vi "Time Trace.vi"() -> ()   [LabVIEW 2011]
uses:
  <vilib>/DAQmx/read.llb/DAQmx Read (Counter U32 1Chan 1Samp).vi
  <vilib>/DAQmx/create/channels.llb/DAQmx Create Channel (CI-Count Edges).vi
  <vilib>/DAQmx/configure/timing.llb/DAQmx Timing (Sample Clock).vi
  <vilib>/DAQmx/miscellaneous.llb/DAQmx Fill In Error Info.vi
  <vilib>/Utility/file.llb/Write To Spreadsheet File (DBL).vi
  Program Files/National Instruments/LabVIEW 2011/resource/objmgr/daqmx.rc
panel:
  in  "Save?":bool
  in  "file path (dialog if empty)":path
  out "XY Graph":cluster{"Y":dbl[], "Y":dbl[]}[](graph)
  in  "Time Target (s)":dbl=1.0
  in  "stop":bool
  in  "rate (Hz)":dbl=1000.0 format="%0.2f"
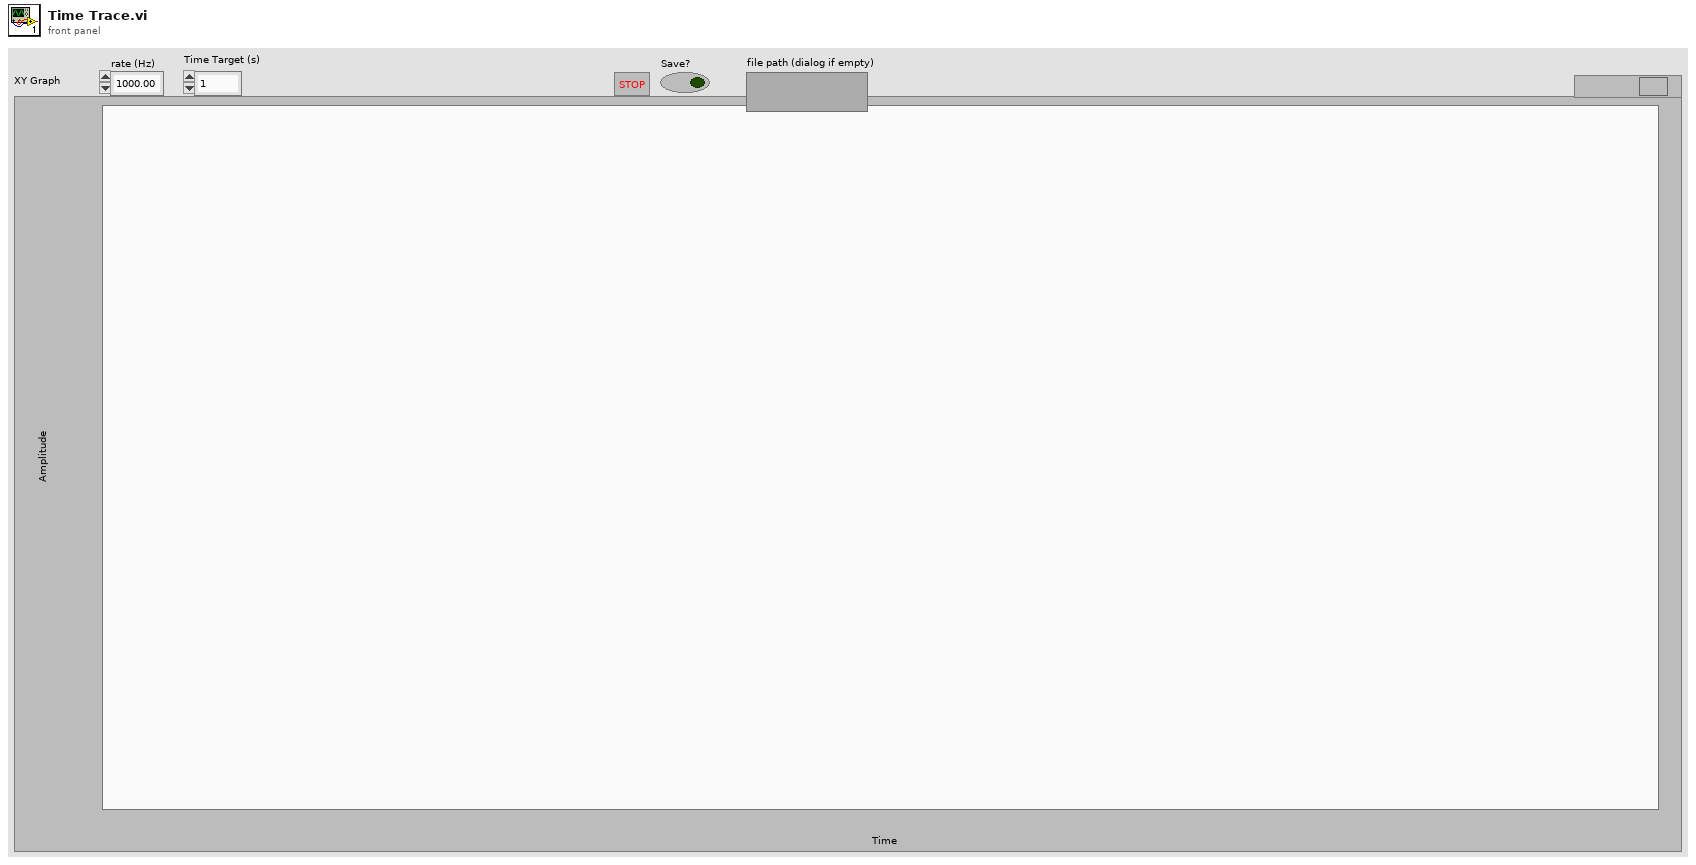
[diagram p1: front panel]
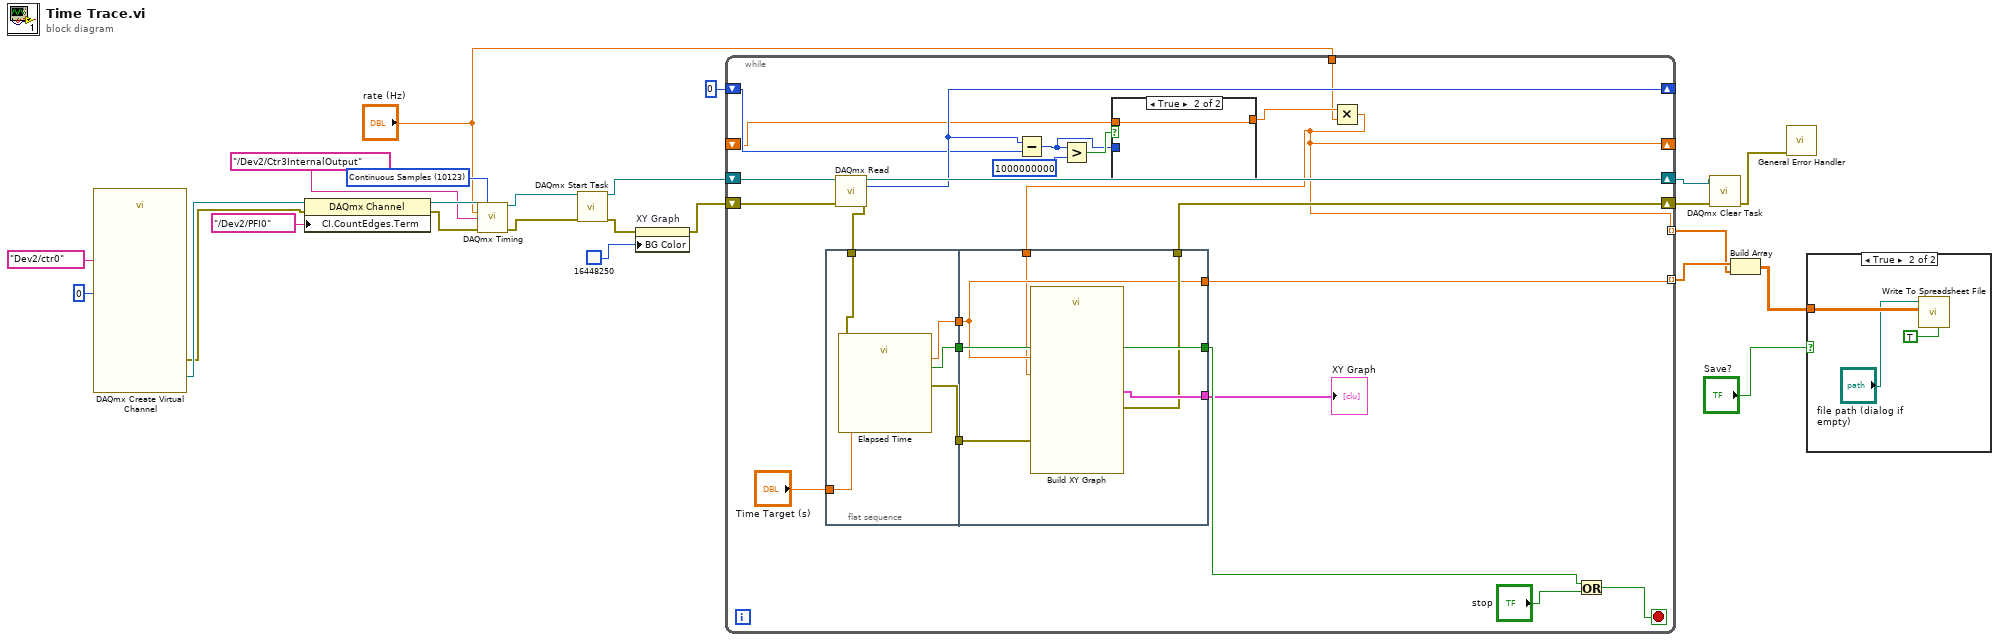
[diagram p0: block diagram]
diagram:
  w4 = 10123 items=["Finite Samples"=10178, "Continuous Samples"=10123, "Hardware Timed Single Point"=12522] ("sample mode")
  n1 = call-poly <vilib>:"DAQmx Create Virtual Channel.vi"("initial count"=u32 0, "counter"=tag "Dev2/ctr0") -> ("task out"=w21:refnum<k21>, "error out"=w20:errorcluster)  [unwired: 6 in, 6 out]
  n2 = property class="DAQmx Channel"(reference=w21, error in=w20, "CI.CountEdges.Term"=tag "/Dev2/PFI0") -> (reference out=w8:refnum<k21>, error out=w7:errorcluster)
  n3 = call-poly <vilib>:"DAQmx Timing.vi"("task/channels in"=w8, "sample mode"=w4, "rate"="rate (Hz)", "source"=tag "/Dev2/Ctr3InternalOutput", "error in"=w7) -> ("task out"=w6:refnum<k21>, "error out"=w5:errorcluster)  [unwired: 9 in]
  n4 = call <vilib>:"DAQmx Start Task.vi"("task/channels in"=w6, "error in"=w5) -> ("task out"=w19:refnum<k21>, "error out"=w12:errorcluster)  [unwired: 12 out]
  n5 = property on="XY Graph" class="XYGraph (strict)"(error in=w12, "BG Color"=u32 16448250) -> (error out=w11:errorcluster)  [unwired: 1 in, 1 out]
  n6 = while {
    shift-right: [w36] -> w17
    shift-left: w11 -> [w44]
    shift-right: [w43] -> w18
    shift-left: w19 -> [w45]
    tunnel: [w34] -> w16 mode=indexing
    shift-right: [w33] -> _
    shift-left: u32 0 ("data") -> [w30]
    tunnel: [w26] -> w13 mode=indexing
    shift-right: [w26] -> _
    shift-left: _ -> [w28]
    tunnel: "rate (Hz)" -> [w25]
    stop <- w46 stop-if-true
    n7 = flat-sequence {
      tunnel: [w54] -> w42
      tunnel: [w50] -> w40
      tunnel: "Time Target (s)" -> [w53]
      tunnel: w38 -> [w52]
      tunnel: [w51] -> w37
      tunnel: [w60] -> w41
      tunnel: w42 -> [w60]
      tunnel: [w59] -> w35
      tunnel: w40 -> [w56]
      tunnel: w37 -> [w58]
      tunnel: [w57] -> w36
      tunnel: [w56] -> w34
      tunnel: w26 -> [w55]
      frame #0 {
        n8 = call "Elapsed Time"("Time Target (s)"=w53, "error in (no error)"=w52) -> ("Elapsed Time (s)"=w50:dbl, "Time has Elapsed"=w54:bool, "error out"=w51:errorcluster)  [unwired: 10 in, 5 out]
      }
      frame #1 {
        n9 = call "Build XY Graph"("error in (no error)"=w58, "Y Input"=w55, "X Input"=w56) -> ("error out"=w57:errorcluster, "XY Graph"=w59:cluster{"Y":dbl[], "Y":dbl[]}[])  [unwired: 2 in, 5 out]
      }
    }
    n10 = call-poly <vilib>:"DAQmx Read.vi"("task/channels in"=w45, "error in"=w44) -> ("task out"=w43:refnum<k21>, "data"=w33:u32, "error out"=w38:errorcluster)  [unwired: 11 in]
    n11 = Subtract(x=w33, y=w30) -> (x-y=w29:u32)
    n12 = Greater?(x=w29, y=u32 1000000000) -> (0:w31:bool)
    n13 = case shown="True" w31 {
      tunnel: w29 -> [w48 _]
      tunnel: [w48 w49] -> w27
      tunnel: w28 -> [_ w49]
      frame False {
      }
      frame True {
      }
    }
    n14 = Multiply(x=w27, y=w25) -> (x*y=w26:dbl)
    n15 = Or(x=w41, y="stop") -> (x .or. y?=w46:bool)
    "XY Graph" <- w35
  }
  n16 = call <vilib>:"DAQmx Clear Task.vi"("task in"=w18, "error in"=w17) -> ("error out"=w14:errorcluster)  [unwired: 13 in]
  n17 = Build Array(w16, w13) -> (w15:dbl[][])
  n18 = call <vilib>:"General Error Handler.vi"("error in (no error)"=w14) -> ()  [unwired: 10 in, 5 out]
  n19 = case shown="True" "Save?" {
    tunnel: w15 -> [_ w63]
    frame False {
    }
    frame True {
      n20 = call-poly <vilib>:"Write To Spreadsheet File.vi"("transpose? (no:F)"=TRUE, "2D data"=w63, "file path (dialog if empty)"="file path (dialog if empty)") -> ()  [unwired: 5 in, 1 out]
    }
  }
